vi "methane.vi"() -> ()   [LabVIEW 2010]
uses:
  TCP DAQ/Send 1 Scan multi-channel.vi
  DAQ configuration/channel identifier.ctl
  support/methane method.ctl
panel:
  in  "Monitor Data":bool
  in  "stop":bool
  in  "Port":cluster{"module":u8, "channel":u8}={"module"=1, "channel"=0} {"channel" max=31; "module" min=1 step=1}
  out "Port Set 2":T1[](array[typedef])
  out "Port Set 1":T1[](array[typedef])
  in  "Tab Control":enum32{"graphs", "configuration"}(tab)=enum."configuration"
  out "Set 2":cluster{dbl[], dbl[]}[](graph)
  out "Set 1":cluster{dbl[], dbl[]}[](graph)
  in  "State":cluster{"Save":bool, "Load":bool}
  in  "Methane Method":T2={"scaling kPa/volt"=1032.0, "module"=1, "data interval (s)"=1, "First channel Set 1"=0, "First channel Set 2"=0, "Sample Set 1"=["", "", "", "", "", "", "", "", "", "", "", "", "", "", "", " "], "Sample Set 2"=["", "", "", "", "", "", "", "", "", "", "", "", "", "", "", " "], "Samples Set 1"=0, "Samples Set2"=0, "history length"=1000, "number Tue"=[], "number Wed"=[]} {"history length" min=1; "data interval (s)" min=1; "module" min=1 step=1}
  in  "update":bool
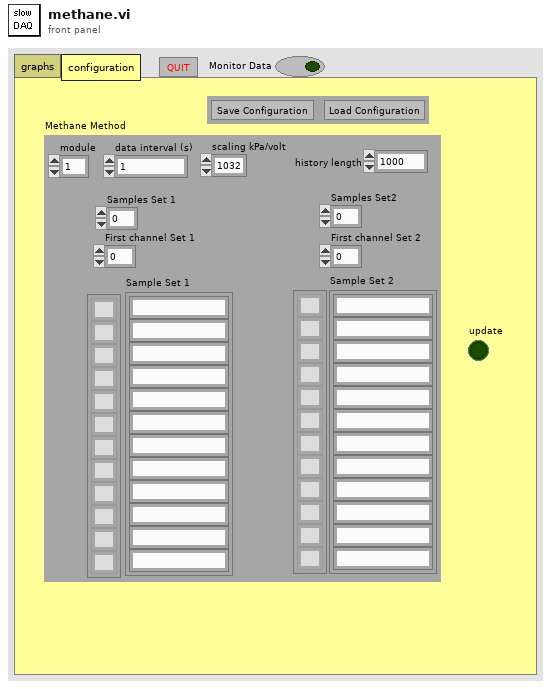
[diagram p1: front panel]
types:
  T1 = typedef "channel identifier.ctl" = u16
  T2 = typedef "methane method.ctl" = cluster{"scaling kPa/volt":dbl, "module":u8, "data interval (s)":i32, "First channel Set 1":i8, "First channel Set 2":i8, "Sample Set 1":string[], "Sample Set 2":string[], "Samples Set 1":i8, "Samples Set2":i8, "history length":u16, "number Tue":string[], "number Wed":string[]}
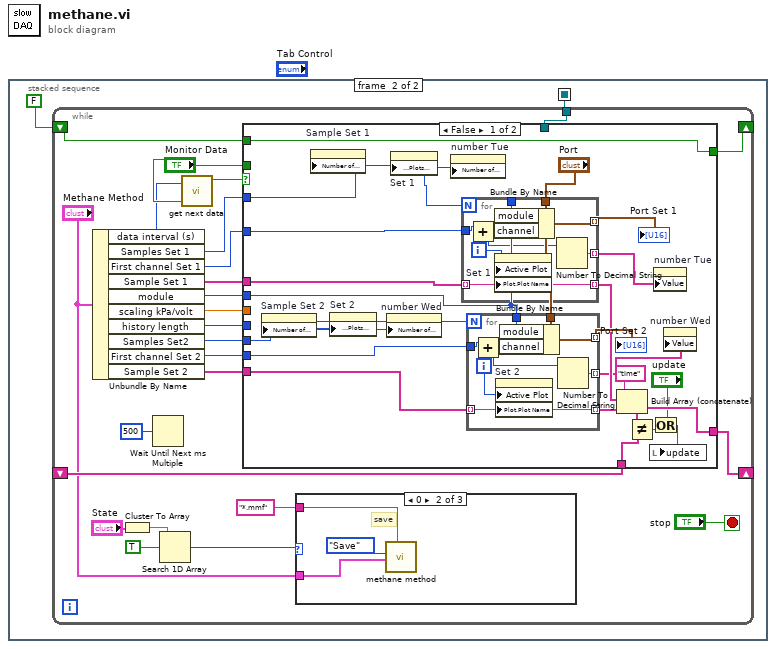
[diagram p0: block diagram]
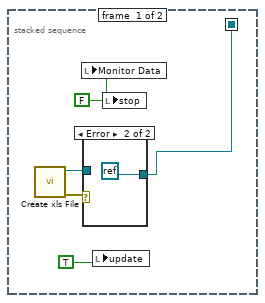
[diagram p2: hidden frame]
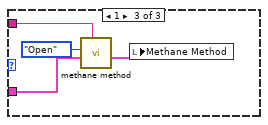
[diagram p5: hidden frame]
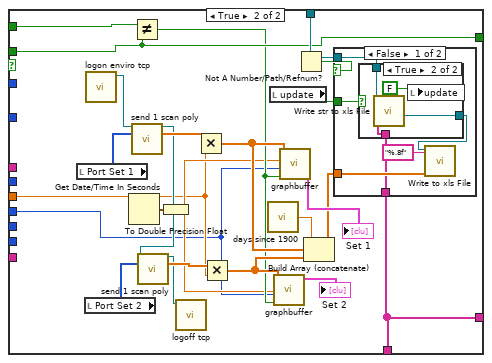
[diagram p6: hidden frame]
diagram:
  n1 = stacked-sequence {
    seq-local: [w4 _] -> [_ w9]
    frame #0 {
      w2 = FALSE ("stop")
      n2 = call "Create xls File.vi"() -> ("error out"=w3:errorcluster, "refnum"=w5:refnum<file>)  [unwired: 4 in, 2 out]
      n3 = local write "Monitor Data"(w2) -> ()
      n4 = case shown="Error" w3 {
        tunnel: w5 -> [w6 _]
        tunnel: [w6 refnum<k0> refnum] -> w4
        frame No Error {
        }
        frame Error {
        }
      }
      n5 = local write "update"(TRUE ("stop")) -> ()
      n6 = local write "stop"(w2) -> ()
    }
    frame #1 {
      n7 = while {
        shift-left: _ -> [w26]
        shift-right: [w27] -> _
        shift-left: FALSE ("Monitor Data") -> [w28]
        shift-right: [w29] -> _
        tunnel: w9 -> [w32]
        stop <- "stop" stop-if-true
        n8 = Unbundle By Name("Methane Method") -> ("data interval (s)"=w23:i32, "Samples Set 1"=w22:i8, "First channel Set 1"=w21:i8, "Sample Set 1"=w17:string[], "module"=w20:u8, "scaling kPa/volt"=w25:dbl, "history length"=w24:u16, "Samples Set2"=w19:i8, "First channel Set 2"=w18:i8, "Sample Set 2"=w16:string[])
        n9 = Cluster To Array(cluster="State") -> (array=w14:bool[])
        n10 = Wait Until Next ms Multiple(millisecond multiple=u32 500) -> ()  [unwired: 1 out]
        n11 = Search 1D Array(1D array=w14, element=TRUE) -> (index of element=w12:i32)  [unwired: 1 in]
        n12 = call "get next data.vi"("Monitor Data"="Monitor Data", "data interval (s)"=w23) -> ("get next"=w31:bool)
        n13 = case shown="False" w31 {
          tunnel: w32 -> [_ w97]
          tunnel: "Monitor Data" -> [_ w87]
          tunnel: [w59 w87] -> w29
          tunnel: w28 -> [w59 w88]
          tunnel: [w55 w84] -> w27
          tunnel: w26 -> [w56 w84]
          tunnel: w25 -> [_ w81]
          tunnel: w24 -> [_ w80]
          tunnel: w22 -> [w50 _]
          tunnel: w21 -> [w49 _]
          tunnel: w20 -> [w48 _]
          tunnel: w19 -> [w47 _]
          tunnel: w18 -> [w46 _]
          tunnel: w17 -> [w45 _]
          tunnel: w16 -> [w44 _]
          frame False {
            n14 = property on="Sample Set 2" class="Arr (strict)"("Number of Rows"=w47) -> ()  [unwired: 2 in, 2 out]
            n15 = property on="Sample Set 1" class="Arr (strict)"("Number of Rows"=w50) -> ()  [unwired: 2 in, 2 out]
            n16 = property on="Set 2" class="XYGraph (strict)"("Legend:Plots Shown"=w47) -> ()  [unwired: 2 in, 2 out]
            n17 = property on="number Wed" class="Arr (strict)"("Number of Rows"=w47) -> ()  [unwired: 2 in, 2 out]
            n18 = property on="Set 1" class="XYGraph (strict)"("Legend:Plots Shown"=w50) -> ()  [unwired: 2 in, 2 out]
            n19 = property on="number Tue" class="Arr (strict)"("Number of Rows"=w50) -> ()  [unwired: 2 in, 2 out]
            n20 = for {
              N: w50 -> [_]
              tunnel: [w72] -> w62 mode=indexing
              tunnel: w48 -> [w78]
              tunnel: w49 -> [w76]
              tunnel: "Port" -> [w75]
              tunnel: w45 -> [w73] mode=indexing
              tunnel: [w73] -> w58 mode=indexing
              tunnel: [w71] -> w43 mode=indexing
              i -> [w74]
              n21 = Add(x=w76, y=w74) -> (x+y=w77:i32)
              n22 = Bundle By Name(cluster=w75, "module"=w78, "channel"=w77) -> (w72:cluster{"module":u8, "channel":u8})
              n23 = property on="Set 1" class="XYGraph (strict)"("Active Plot"=w74, "Plot.Plot Name"=w73) -> ()  [unwired: 2 in, 2 out]
              n24 = Number To Decimal String(number=w77) -> (decimal integer string=w71:string)  [unwired: 1 in]
            }
            "Port Set 1" <- w62
            n25 = for {
              N: w47 -> [_]
              tunnel: [w70] -> w60 mode=indexing
              tunnel: w48 -> [w69]
              tunnel: w46 -> [w66]
              tunnel: "Port" -> [w65]
              tunnel: w44 -> [w64] mode=indexing
              tunnel: [w64] -> w57 mode=indexing
              tunnel: [w63] -> w42 mode=indexing
              i -> [w68]
              n26 = Add(x=w66, y=w68) -> (x+y=w67:i32)
              n27 = property on="Set 2" class="XYGraph (strict)"("Active Plot"=w68, "Plot.Plot Name"=w64) -> ()  [unwired: 2 in, 2 out]
              n28 = Bundle By Name(cluster=w65, "module"=w69, "channel"=w67) -> (w70:cluster{"module":u8, "channel":u8})
              n29 = Number To Decimal String(number=w67) -> (decimal integer string=w63:string)  [unwired: 1 in]
            }
            "Port Set 2" <- w60
            n30 = Build Array (concatenate)("time", w58, w57) -> (w55:string[])
            n31 = Not Equal?(x=w55, y=w56) -> (x != y?=w53:bool)
            n32 = Or(x="update", y=w53) -> (x .or. y?=w52:bool)
            n33 = local write "update"(w52) -> ()
            n34 = property on="number Tue" class="Arr (strict)"("Value"=w43) -> ()  [unwired: 2 in, 2 out]
            n35 = property on="number Wed" class="Arr (strict)"("Value"=w42) -> ()  [unwired: 2 in, 2 out]
          }
          frame True {
            n36 = local read "Port Set 1"() -> (w96:T1[])
            n37 = local read "Port Set 2"() -> (w95:T1[])
            n38 = call "logon enviro tcp.vi"() -> ("connection ID"=w100:refnum<k5>)  [unwired: 9 in, 2 out]
            n39 = Get Date/Time In Seconds() -> (seconds since 1Jan1904=w79:timestamp)
            n40 = Not Equal?(x=w88, y=w87) -> (x != y?=w86:bool)
            n41 = call-poly "send 1 scan poly.vi"("Connection ID in"=w100, "Channel"=w96) -> ("Connection ID out"=w99:refnum<k5>, "voltage data"=w102:sgl[])  [unwired: 6 in, 6 out]
            n42 = call-poly "send 1 scan poly.vi"("Connection ID in"=w99, "Channel"=w95) -> ("Connection ID out"=w89:refnum<k5>, "voltage data"=w94:sgl[])  [unwired: 6 in, 6 out]
            n43 = To Double Precision Float(number=w79) -> (double precision float=w82:dbl)
            n44 = call "logoff tcp.vi"("Connection ID"=w89) -> ()  [unwired: 9 in, 2 out]
            n45 = Multiply(x=w102, y=w81) -> (x*y=w92:dbl[])
            n46 = Multiply(x=w94, y=w81) -> (x*y=w93:dbl[])
            n47 = call "days since 1900.vi"() -> ("Days"=w83:dbl)  [unwired: 1 in]
            n48 = local read "update"() -> (w85:bool)
            n49 = call "graphbuffer.vi"("Reset"=w86, "history length"=w80, "Time"=w82, "data"=w93) -> ("Multiplot graph data"=→"Set 2":cluster{dbl[], dbl[]}[])  [unwired: 5 in, 2 out]
            n50 = call "graphbuffer.vi"("Reset"=w86, "history length"=w80, "Time"=w82, "data"=w92) -> ("Multiplot graph data"=→"Set 1":cluster{dbl[], dbl[]}[])  [unwired: 5 in, 2 out]
            n51 = Not A Number/Path/Refnum?(number/path/refnum=w97) -> (NaN/Path/Refnum?=w98:bool)
            n52 = Build Array (concatenate)(w83, w92, w93) -> (w91:dbl[])
            n53 = case shown="False" w98 {
              tunnel: w97 -> [w105 _]
              tunnel: w91 -> [w108 _]
              tunnel: w85 -> [w107 _]
              tunnel: w84 -> [w104 _]
              frame False {
                n54 = case shown="True" w107 {
                  tunnel: w105 -> [w109 w113]
                  tunnel: [w109 w112] -> w106
                  tunnel: w104 -> [_ w110]
                  frame False {
                  }
                  frame True {
                    n55 = call "Write str to xls File.vi"("error in (no error)"=w110, "refnum"=w113) -> ("dup refnum"=w112:refnum<file>)  [unwired: 8 in, 1 out]
                    n56 = local write "update"(FALSE ("update")) -> ()
                  }
                }
                n57 = call "Write to xls File.vi"("format (%.3f)"="%.8f", "error in (no error)"=w108, "refnum"=w106) -> ()  [unwired: 7 in, 2 out]
              }
              frame True {
              }
            }
          }
        }
        n58 = case shown="0" w12 {
          tunnel: "Methane Method" -> [_ w37 w40]
          tunnel: "*.mmf" ("pattern") -> [_ w35 w38]
          frame -1, Default {
          }
          frame 0 {
            # "save"
            n59 = call "methane method.vi"("pattern"=w35, "data in"=w37, "Action"=enum16{"Save", "Open"}."Save") -> ()  [unwired: 7 in, 2 out]
          }
          frame 1 {
            n60 = call "methane method.vi"("pattern"=w38, "data in"=w40, "Action"=enum16{"Save", "Open"}."Open") -> ("data out"=w39:T2)  [unwired: 7 in, 1 out]
            n61 = local write "Methane Method"(w39) -> ()
          }
        }
      }
    }
  }
